vi "Read String Config.vi"(8 "error in (no error)":errorcluster, 11 "RxTxCamera in":refnum<class "RxTxCamera.lvclass">) -> (0 "error out":errorcluster, 2 "Camera Setup":T1={"Acquisition Mode"=1, "Read Mode"=4, "Trigger"=0, "Conventional/EM"=0, "Shutter Mode"=2, "Shutter TTL"=0, "Time to open Shutter"=50, "Time to close Shutter"=50, "Exposure time"=0.0, "Readout Rate"=0, "VShift Speed"=0, "Pre amp"=0, "Initial line"=1, "Initial column"=1, "Final column"=1024, "Final line"=1024, "hbin"=1, "vbin"=1, "Temperature"=20.0, "Cooler ON/OFF"=0, "FITS Format"=0, "tiff position"=1, "Tiff Type"=0, "Image Format"="", "Image Path"=""} {"Tiff Type" items=["8-bit", "16-bit", "Color"]; "FITS Format" items=["Unsigned 16", "Unsigned 32", "Signed 16", "Signed 32", "Float"]; "Cooler ON/OFF" items=["Cooler OFF", "Cooler ON"]; "Shutter TTL" items=["TTL Low", "TTL High"]; "Shutter Mode" items=["Fully Auto", "OPEN", "CLOSED"]; "Conventional/EM" items=["Conventional", "EM Gain"]; "Trigger" items=["Internal", "External", "N/A", "N/A", "N/A", "N/A", "External Start", "External Exposure (bulb)", "N/A", "External FVB EM", "Software", "N/A", "External Charge Shifting"]; "Read Mode" items=["Full Vertical Binning", "Multi-Track", "Random-Track", "Single-Track", "Image"]; "Acquisition Mode" items=["RESERVED", "Single Scan", "Accumulate", "Kinetics", "Fast Kinetics", "Run Til Abort", "RESERVED", "RESERVED", "RESERVED", "RESERVED", "Time Delayed Integration"]}, 3 "RxTxCamera out":refnum<class "RxTxCamera.lvclass">)   [LabVIEW 2018, in "RxTxCamera.lvclass"]
doc: "Este VI realiza a leitura da string de configuração da câmera, retornando um cluster contendo as informações de configuração."
uses:
  RxTxCamera.lvclass
  C:/Users/Cliente/Desktop/Software Echarpe/RxTx/RxTx.lvclass
  RxTxCamera.lvclass/RxTxCamera.ctl
  RxTx/RxTx.lvclass/RxTx.ctl
  Construct String Setup Cam/Construct String Setup Cam.lvclass
  RxTx/RxTx.lvclass
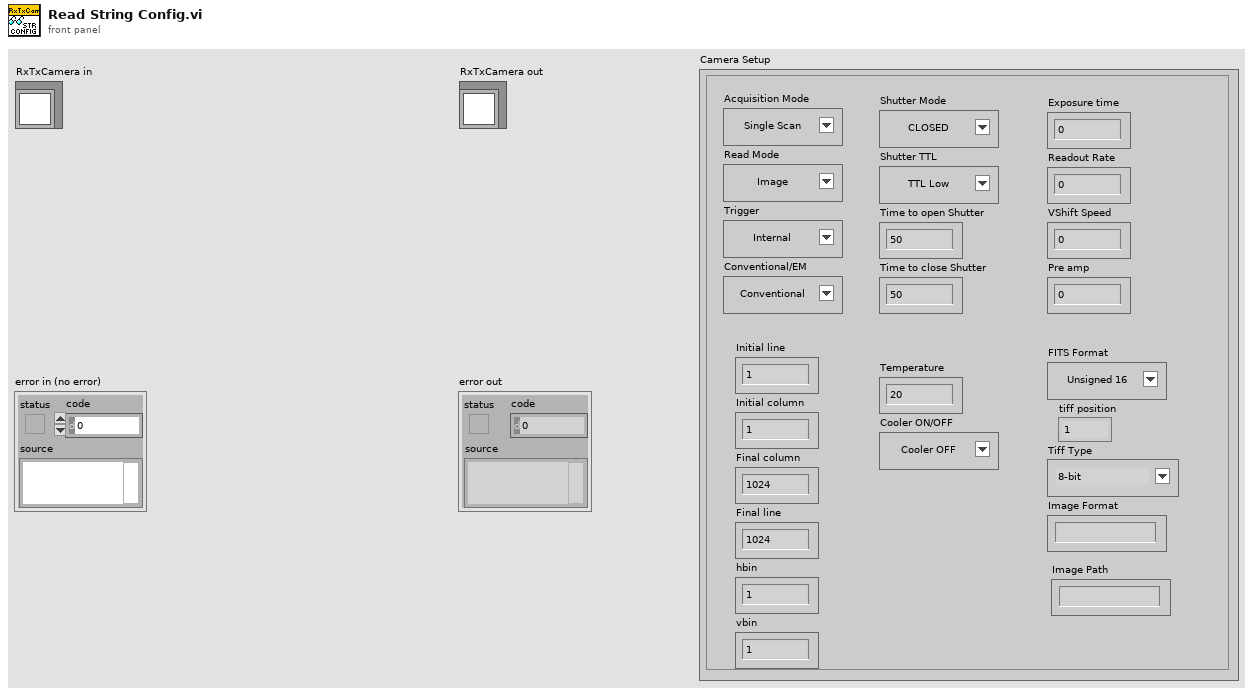
[diagram p1: front panel]
types:
  T1 = cluster{"Acquisition Mode":u16, "Read Mode":u16, "Trigger":u16, "Conventional/EM":u16, "Shutter Mode":u16, "Shutter TTL":u16, "Time to open Shutter":u16, "Time to close Shutter":u16, "Exposure time":dbl, "Readout Rate":u16, "VShift Speed":u16, "Pre amp":u16, "Initial line":u16, "Initial column":u16, "Final column":u32, "Final line":u32, "hbin":u16, "vbin":u16, "Temperature":dbl, "Cooler ON/OFF":u16, "FITS Format":u16, "tiff position":u16, "Tiff Type":u16, "Image Format":string, "Image Path":string}
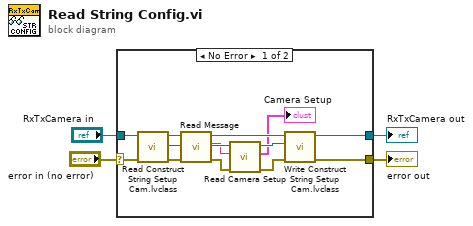
[diagram p0: block diagram]
diagram:
  n1 = case shown="No Error" "error in (no error)" {
    selector: "error in (no error)" -> [w7 w18]
    tunnel: [w16 w18] -> w3
    tunnel: [w17 w19] -> w1
    tunnel: "RxTxCamera in" -> [w6 w19]
    frame No Error {
      n2 = call "Read Construct String Setup Cam.lvclass.vi"("error in (no error)"=w7, "RxTxCamera in"=w6) -> ("error out"=w11:errorcluster, "Construct String Setup Cam.lvclass"=w14:refnum<class "Construct String Setup Cam.lvclass">, "RxTxCamera out"=w9:refnum<class "RxTxCamera.lvclass">)  [unwired: 7 in]
      n3 = call "Read Message.vi"("error in (no error)"=w11, "RxTx in"=w9) -> ("error out"=w10:errorcluster, "Message"=w12:string, "RxTx out"=w8:refnum<class "RxTxCamera.lvclass">)  [unwired: 7 in]
      n4 = call "Read Camera Setup.vi"("error in (no error)"=w10, "String Camera Setup"=w12, "Construct String Setup Cam in"=w14) -> ("error out"=w15:errorcluster, "Camera Setup"=→"Camera Setup":T1, "Construct String Setup Cam out"=w13:refnum<class "Construct String Setup Cam.lvclass">)  [unwired: 6 in]
      n5 = call "Write Construct String Setup Cam.lvclass.vi"("error in (no error)"=w15, "Construct String Setup Cam.lvclass"=w13, "RxTxCamera in"=w8) -> ("error out"=w16:errorcluster, "RxTxCamera out"=w17:refnum<class "RxTxCamera.lvclass">)  [unwired: 7 in]
    }
    frame Error {
    }
  }
  "error out" <- w3
  "RxTxCamera out" <- w1
